vi "SetupConvertTreeToSetupObj.vi"(8 "error in (no error)":errorcluster, 11 "TreeControl in":refnum<vi>) -> (0 "error out":errorcluster, 3 "Setup out":refnum<class "Setup.lvclass">)   [LabVIEW 2013, in "DataCreation.lvlib"]
uses:
  DataCreation.lvlib
  classes/Datastructure/Setup/Setup.lvclass
  classes/Datastructure/Image/img.lvclass
  classes/Datastructure/Device/Device.lvclass
  <vilib>/regexp/Match Regular Expression.xnode
panel:
  out "whole match":string
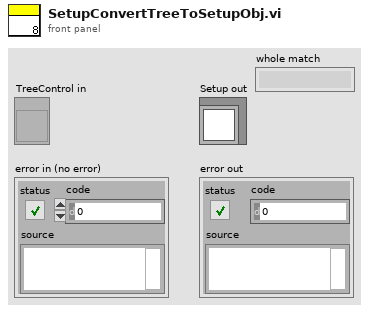
[diagram p1: front panel]
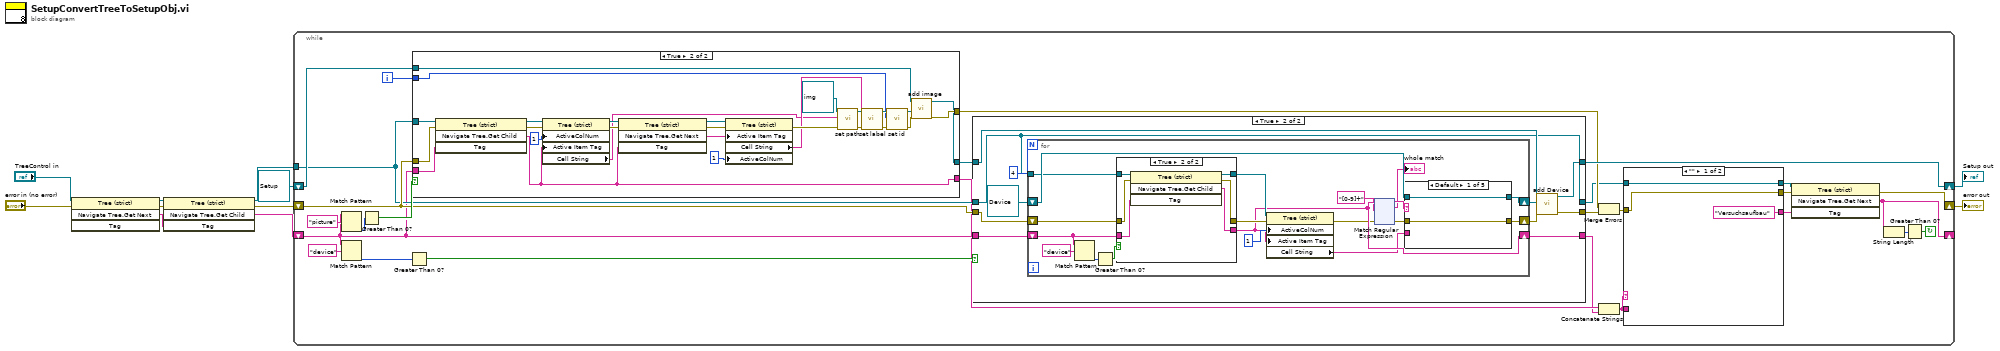
[diagram p0: block diagram]
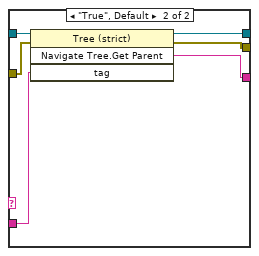
[diagram p2: hidden frame]
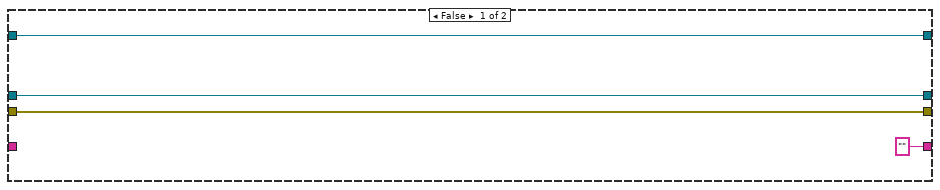
[diagram p3: hidden frame]
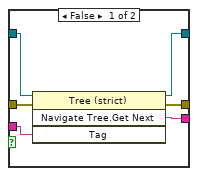
[diagram p4: hidden frame]
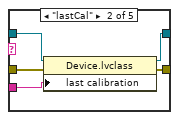
[diagram p5: hidden frame]
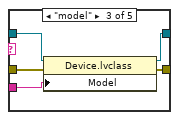
[diagram p6: hidden frame]
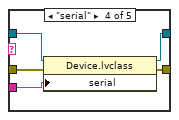
[diagram p7: hidden frame]
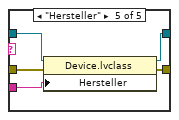
[diagram p8: hidden frame]
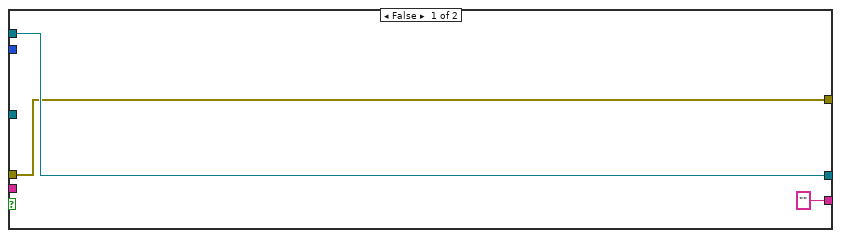
[diagram p9: hidden frame]
diagram:
  n1 = invoke class="Tree (strict)" method="Navigate Tree.Get Next"(reference="TreeControl in", error in="error in (no error)") -> (reference out=w5:refnum<vi>, error out=w6:errorcluster, "Navigate Tree:Get Next Item"=w7:string)  [unwired: 2 in, 1 out]
  n2 = invoke class="Tree (strict)" method="Navigate Tree.Get Child"(reference=w5, error in=w6, "Tag"=w7) -> (reference out=w10:refnum<vi>, error out=w8:errorcluster, "Navigate Tree:Get Child"=w9:string)  [unwired: 1 in, 1 out]
  n3 = while {
    shift-right: [w16] -> w1
    shift-left: w8 -> [w32]
    shift-right: [w25] -> w2
    shift-left: refnum<class "Setup.lvclass"> refnum ("Setup Ausgang") -> [w31]
    shift-right: [w14] -> _
    shift-left: w9 -> [w29]
    tunnel: w10 -> [w30]
    i -> [w12]
    stop <- w19 continue-if-true
    n4 = Match Pattern(string=w29, regular expression="picture" ("Regulärer Ausdruck")) -> (offset past match=w37:i32)  [unwired: 1 in, 3 out]
    n5 = Match Pattern(string=w29, regular expression="device" ("Regulärer Ausdruck")) -> (offset past match=w33:i32)  [unwired: 1 in, 3 out]
    n6 = Greater Than 0?(x=w37) -> (x > 0?=w36:bool)
    n7 = Greater Than 0?(x=w33) -> (x > 0?=w35:bool)
    n8 = case shown="True" w36 {
      tunnel: w29 -> [_ w240]
      tunnel: w32 -> [w230 w241]
      tunnel: w30 -> [_ w242]
      tunnel: [w230 w246] -> w24
      tunnel: w31 -> [w231 w245]
      tunnel: [w231 w239] -> w26
      tunnel: ["" ("Navigate Tree:Get Child") w238] -> w28
      tunnel: w12 -> [_ w235]
      frame False {
      }
      frame True {
        n9 = invoke class="Tree (strict)" method="Navigate Tree.Get Child"(reference=w242, error in=w241, "Tag"=w240) -> (reference out=w244:refnum<vi>, error out=w243:errorcluster, "Navigate Tree:Get Child"=w238:string)  [unwired: 1 in, 1 out]
        n10 = property class="Tree (strict)"(reference=w244, error in=w243, "ActiveColNum"=1 ("Active Cell:Active Column Number"), "Active Item Tag"=w238) -> (reference out=w254:refnum<vi>, error out=w255:errorcluster, "Cell String"=w250:string)
        n11 = invoke class="Tree (strict)" method="Navigate Tree.Get Next"(reference=w254, error in=w255, "Tag"=w238) -> (reference out=w253:refnum<vi>, error out=w252:errorcluster, "Navigate Tree:Get Next Item"=w249:string)  [unwired: 1 in, 1 out]
        n12 = property class="Tree (strict)"(reference=w253, error in=w252, "Active Item Tag"=w249, "ActiveColNum"=1 ("Active Cell:Active Column Number")) -> (error out=w259:errorcluster, "Cell String"=w251:string)  [unwired: 1 out]
        n13 = call-dynamic "set path.vi"("error in (no error)"=w259, "path"=w250, "img (Eingang)"=refnum<class "img.lvclass"> refnum ("img.lvclass")) -> ("error out"=w258:errorcluster, "img (Ausgang)"=w256:refnum<class "img.lvclass">)  [unwired: 7 in]
        n14 = call-dynamic "set label.vi"("error in (no error)"=w258, "label"=w251, "img (Eingang)"=w256) -> ("error out"=w236:errorcluster, "img (Ausgang)"=w237:refnum<class "img.lvclass">)  [unwired: 7 in]
        n15 = call-dynamic "set id.vi"("error in (no error)"=w236, "id"=w235, "img in"=w237) -> ("error out"=w234:errorcluster, "img out"=w233:refnum<class "img.lvclass">)  [unwired: 7 in]
        n16 = call-dynamic "add image.vi"("error in (no error)"=w234, "img.lvclass"=w233, "Setup (Eingang)"=w245) -> ("error out"=w246:errorcluster, "Setup (Ausgang)"=w239:refnum<class "Setup.lvclass">)  [unwired: 7 in]
      }
    }
    n17 = case shown="True" w35 {
      tunnel: w32 -> [w49 w54]
      tunnel: w30 -> [w48 w52]
      tunnel: w29 -> [_ w53]
      tunnel: ["" ("Navigate Tree:Get Next Item") w57] -> w27
      tunnel: w26 -> [w50 w61]
      tunnel: [w49 w62] -> w23
      tunnel: [w50 w60] -> w25
      tunnel: [w48 w52] -> w21
      frame False {
      }
      frame True {
        n18 = for {
          N: 4 -> [_]
          shift-right: [w76] -> w57
          shift-left: w53 -> [w63]
          shift-right: [w70] -> w55
          shift-left: refnum<class "Device.lvclass"> refnum ("Device.lvclass") -> [w77]
          shift-right: [w71] -> w56
          shift-left: w54 -> [w78]
          tunnel: w52 -> [w68]
          n19 = Match Pattern(string=w63, regular expression="device") -> (offset past match=w65:i32)  [unwired: 1 in, 3 out]
          n20 = Greater Than 0?(x=w65) -> (x > 0?=w64:bool)
          n21 = case shown="True" w64 {
            tunnel: [w87 w93] -> w81
            tunnel: [w86 w92] -> w80
            tunnel: w63 -> [w84 w91]
            tunnel: w78 -> [w83 w90]
            tunnel: [w85 w89] -> w76
            tunnel: w68 -> [w82 w88]
            frame False {
              n22 = invoke class="Tree (strict)" method="Navigate Tree.Get Next"(reference=w82, error in=w83, "Tag"=w84) -> (reference out=w87:refnum<vi>, error out=w86:errorcluster, "Navigate Tree:Get Next Item"=w85:string)  [unwired: 1 in, 1 out]
            }
            frame True {
              n23 = invoke class="Tree (strict)" method="Navigate Tree.Get Child"(reference=w88, error in=w90, "Tag"=w91) -> (reference out=w93:refnum<vi>, error out=w92:errorcluster, "Navigate Tree:Get Child"=w89:string)  [unwired: 1 in, 1 out]
            }
          }
          n24 = property class="Tree (strict)"(reference=w81, error in=w80, "ActiveColNum"=1 ("Active Cell:Active Column Number"), "Active Item Tag"=w76) -> (error out=w73:errorcluster, "Cell String"=w69:string)  [unwired: 1 out]
          n25 = xnode "Match Regular Expression"("input string"=w76, "regular expression"="[0-9]+", "error in"=w73) -> ("before match"=w75:string, "whole match"=→"whole match":string, "error out"=w72:errorcluster)  [unwired: 3 in, 2 out]
          n26 = case shown="Default" w75 {
            tunnel: w77 -> [w209 w213 w218 w223 w229]
            tunnel: w72 -> [w208 w210 w215 w220 w228]
            tunnel: [w208 w214 w219 w224 w227] -> w71
            tunnel: [w209 w212 w217 w222 w225] -> w70
            tunnel: w69 -> [_ w211 w216 w221 w226]
            frame Default {
            }
            frame "lastCal" {
              n27 = property class="Device.lvclass"(reference=w213, error in=w210, "last calibration"=w211) -> (reference out=w212:refnum<class "Device.lvclass">, error out=w214:errorcluster)
            }
            frame "model" {
              n28 = property class="Device.lvclass"(reference=w218, error in=w215, "Model"=w216) -> (reference out=w217:refnum<class "Device.lvclass">, error out=w219:errorcluster)
            }
            frame "serial" {
              n29 = property class="Device.lvclass"(reference=w223, error in=w220, "serial"=w221) -> (reference out=w222:refnum<class "Device.lvclass">, error out=w224:errorcluster)
            }
            frame "Hersteller" {
              n30 = property class="Device.lvclass"(reference=w229, error in=w228, "Hersteller"=w226) -> (reference out=w225:refnum<class "Device.lvclass">, error out=w227:errorcluster)
            }
          }
        }
        n31 = call-dynamic "add Device.vi"("error in (no error)"=w56, "Device.lvclass"=w55, "Setup Eingang"=w61) -> ("error out"=w62:errorcluster, "Setup Ausgang"=w60:refnum<class "Setup.lvclass">)  [unwired: 7 in]
      }
    }
    n32 = Merge Errors(w24, w23) -> (w22:errorcluster)
    n33 = Concatenate Strings(w28, w27) -> (w13:string)
    n34 = case shown="\"\"" w13 {
      tunnel: w22 -> [w41 w47]
      tunnel: w21 -> [w40 w46]
      tunnel: w13 -> [_ w45]
      tunnel: [w41 w44] -> w18
      tunnel: [w40 w43] -> w17
      tunnel: ["Versuchsaufbau" ("Navigate Tree:Get Parent") w42] -> w15
      frame "" {
      }
      frame "True", Default {
        n35 = invoke class="Tree (strict)" method="Navigate Tree.Get Parent"(reference=w46, error in=w47, "tag"=w45) -> (reference out=w43:refnum<vi>, error out=w44:errorcluster, "Navigate Tree:Get Parent"=w42:string)  [unwired: 1 in, 1 out]
      }
    }
    n36 = invoke class="Tree (strict)" method="Navigate Tree.Get Next"(reference=w17, error in=w18, "Tag"=w15) -> (error out=w16:errorcluster, "Navigate Tree:Get Next Item"=w14:string)  [unwired: 1 in, 2 out]
    n37 = String Length(string=w14) -> (length=w20:i32)
    n38 = Greater Than 0?(x=w20) -> (x > 0?=w19:bool)
  }
  "Setup out" <- w2
  "error out" <- w1
